vi "main(Test DQMH modules).vi"() -> ()   [LabVIEW 2018, in "Application.lvlib"]
uses:
  Application.lvlib
  eMIC response.ctl
  DRV stand.ctl
  type defs/HW config.ctl
  eMICs Cluster.ctl
  SubVIs/App state data.ctl
  SubVIs/Trigger cluster.ctl
  type defs/DMM all config cluster.ctl
  type defs/DMM config cluster.ctl
  SubVIs/FGV DRV data.ctl
  SubVIs/DUT data Mode.ctl
  Instrument Drivers/LV_driver_MBrelay/type defs/FGV enum.ctl
  SubVIs/Step data.ctl
  DRV cluster 2.ctl
  <vilib>/ErrorRing/Error Ring.xnode
  Switches Module/MB switches Module.lvlib
  MB 01 switches Module/MB 01 switches Module.lvlib
  DMM Module/DMM Module.lvlib
  v2_CE14/CE14_v2.lvlib
  Instrument Drivers/LV_driver_MBrelay/MB Relay.lvlib
panel:
  out "PCB":string
  out "Report file Name":string
  in  "RE_Test":bool caption="Again"
  in  "milliseconds to wait":u32=1500
  in  "Log report":bool
  in  "10-1 delay":u32=70
  in  "6_1 delay2":u32=70
  in  "DMM delay":u32=10
  in  "6_1 delay":u32=150
  in  "1-10delay":u32=70
  in  "eMIC delay":u32=70
  in  "DRV number":u8=1 max=60
  in  "Test Single DRV":bool
  in  "Enum":T1(ring)=enum."Fixxed"
  out "Name":string
  out "SAP ID":string
  out "Progress":string
  out "DRV stand":T2
  in  "Auto/Man":bool
  out "DC Measure Completed":bool caption="DC Completed"
  in  "Test Channel 10":bool
  in  "Test Channel 9":bool
  in  "Test Channel 8":bool
  in  "Test Channel 7":bool
  in  "Test Channel 6":bool
  in  "Test Channel 5":bool
  in  "Test Channel 4":bool
  in  "Test Channel 3":bool
  in  "Test Channel 2":bool
  in  "Test Channel 1":bool
  in  "Shorted Circuits Test":bool
  out "CE14  Module did it":bool[](array[boolean])
  out "time elased(ms)":u32
  out "Inst. 9":bool
  in  "Exit":bool
  out "Inst. 8":bool
  out "Inst. 7":bool
  out "Inst. 6":bool
  out "Inst. 5":bool
  out "Inst. 4":bool
  out "Inst. 3":bool
  out "Inst. 2":bool
  out "Inst. 1":bool
  out "new Trigger?":bool
  out "last Trigger?":bool
  out "error out":errorcluster
  out "State log":string
  out "AC  Completed":bool caption="AC Completed"
  in  "Select CE14 eMIC Module Instance":i32(ring)=-1 items=["All"=-1, "1"=1, "2"=2, "3"=3, "4"=4, "5"=5, "6"=6]
  out "New board?":bool
  in  "Test":bool caption="Again"
  out "DRV 61":u32(colorbox)
  in  "Settings":bool
  in  "VIEW":bool caption="Again"
  out "DRV 60":u32(colorbox) caption="60"
  out "DRV 59":u32(colorbox) caption="59"
  out "DRV 58":u32(colorbox) caption="58"
  out "DRV 57":u32(colorbox) caption="57"
  out "DRV 56":u32(colorbox) caption="56"
  out "DRV 55":u32(colorbox) caption="55"
  out "DRV 54":u32(colorbox) caption="54"
  out "DRV 53":u32(colorbox) caption="53"
  out "DRV 52":u32(colorbox) caption="52"
  out "DRV 51":u32(colorbox) caption="51"
  out "DRV 50":u32(colorbox) caption="50"
  out "DRV 49":u32(colorbox) caption="49"
  out "DRV 48":u32(colorbox) caption="48"
  out "DRV 47":u32(colorbox) caption="47"
  out "DRV 46":u32(colorbox) caption="46"
  out "DRV 45":u32(colorbox) caption="45"
  out "DRV 44":u32(colorbox) caption="44"
  out "DRV 43":u32(colorbox) caption="43"
  out "DRV 42":u32(colorbox) caption="42"
  out "DRV 41":u32(colorbox) caption="41"
  out "DRV 40":u32(colorbox) caption="40"
  out "DRV 39":u32(colorbox) caption="39"
  out "DRV 38":u32(colorbox) caption="38"
  out "DRV 37":u32(colorbox) caption="37"
  out "DRV 36":u32(colorbox) caption="36"
  out "DRV 35":u32(colorbox) caption="35"
  out "DRV 34":u32(colorbox) caption="34"
  out "DRV 33":u32(colorbox) caption="33"
  out "DRV 32":u32(colorbox) caption="32"
  out "DRV 31":u32(colorbox) caption="31"
  out "DRV 30":u32(colorbox) caption="30"
  out "DRV 29":u32(colorbox) caption="29"
  out "DRV 28":u32(colorbox) caption="28"
  out "DRV 27":u32(colorbox) caption="27"
  out "DRV 26":u32(colorbox) caption="26"
  out "DRV 25":u32(colorbox) caption="25"
  out "DRV 24":u32(colorbox) caption="24"
  out "DRV 23":u32(colorbox) caption="23"
  out "DRV 22":u32(colorbox) caption="22"
  out "DRV 21":u32(colorbox) caption="21"
  out "DRV 20":u32(colorbox) caption="20"
  out "DRV 19":u32(colorbox) caption="19"
  out "DRV 18":u32(colorbox) caption="18"
  out "DRV 17":u32(colorbox) caption="17"
  out "DRV 16":u32(colorbox) caption="16"
  out "DRV 15":u32(colorbox) caption="15"
  out "DRV 14":u32(colorbox) caption="14"
  out "DRV 13":u32(colorbox) caption="13"
  out "DRV 12":u32(colorbox) caption="12"
  out "DRV 11":u32(colorbox) caption="11"
  out "DRV 10":u32(colorbox) caption="10"
  out "DRV 9":u32(colorbox) caption="9"
  out "DRV 8":u32(colorbox) caption="8"
  out "DRV 7":u32(colorbox) caption="7"
  out "DRV 6":u32(colorbox) caption="6"
  out "DRV 5":u32(colorbox) caption="5"
  out "DRV 4":u32(colorbox) caption="4"
  out "DRV 3":u32(colorbox) caption="3"
  out "DRV 2":u32(colorbox) caption="2"
  out "DRV 1":u32(colorbox) caption="1"
  out "version":string caption="Version"
  out "Module ID":i32
  in  "Tab Control":T3(tab)
  out "Short DRV":bool[][](array[boolean])
  in  "Mux 10-1":bool
  in  "mux 6-1":bool
  in  "Read Optos":bool
  in  "Select DMM's Current Input":bool
  in  "mux2-1(DMM I) encode":enum16{"DMM I (0.5)", "DMM I (12)"}(ring)
  in  "mux 6-1 data":T4(ring)
  in  "mux 10-1 data":T5(ring)
  in  "set value":bool
  in  "Set trigger value":bool
  out "trigger Value":bool
  in  "Read trigger":bool
  in  "Reset JIG":bool
  in  "eMIC":bool
  in  "DEMUX 1-10":bool
  in  "TurnON/OFF +5V":bool
  in  "5V Value":bool
  in  "demux1_10(x6)_encode":T6(ring)
  in  "eMIC 6 values":bool[](array[boolean])=[FALSE, FALSE, FALSE, FALSE, FALSE, FALSE]
  in  "DMM query":bool
  in  "connect DMM":bool
  in  "DMM read dual value":bool
  in  "config DMM":bool
  in  "Detector Rate":u8(ring)=2 items=["SLOW", "MID", "FAST"]
  in  "DCI range":dbl=0.5
  in  "DCV range":dbl=1000.0
  out "DCV(Volts)":dbl
  out "DCI(mA)":dbl
  out "DMM func?":string
  out "DMM range?":string
  in  "request AC-all":bool
  in  "Open COM eMIC":bool
  in  "check connected":bool
  out "eMIC 1":T7
  out "eMIC 2":T7
  out "eMIC 3":T7
  out "eMIC 4":T7
  out "eMIC 5":T7
  out "eMIC 6":T7
  out "EMIC connected":bool[](array[boolean])
  out "AC switches Module":bool
  out "DC Measure Module":bool
  out "DC Switches Module":bool
  out "AC Measure Module":bool
  # "HV-60D: ON-LINE TESTER FOR LED POWER DRIVER"
  # "60"
  # "6"
  # "12"
  # "18"
  # "24"
  # "30"
  # "36"
  # "42"
  # "48"
  # "54"
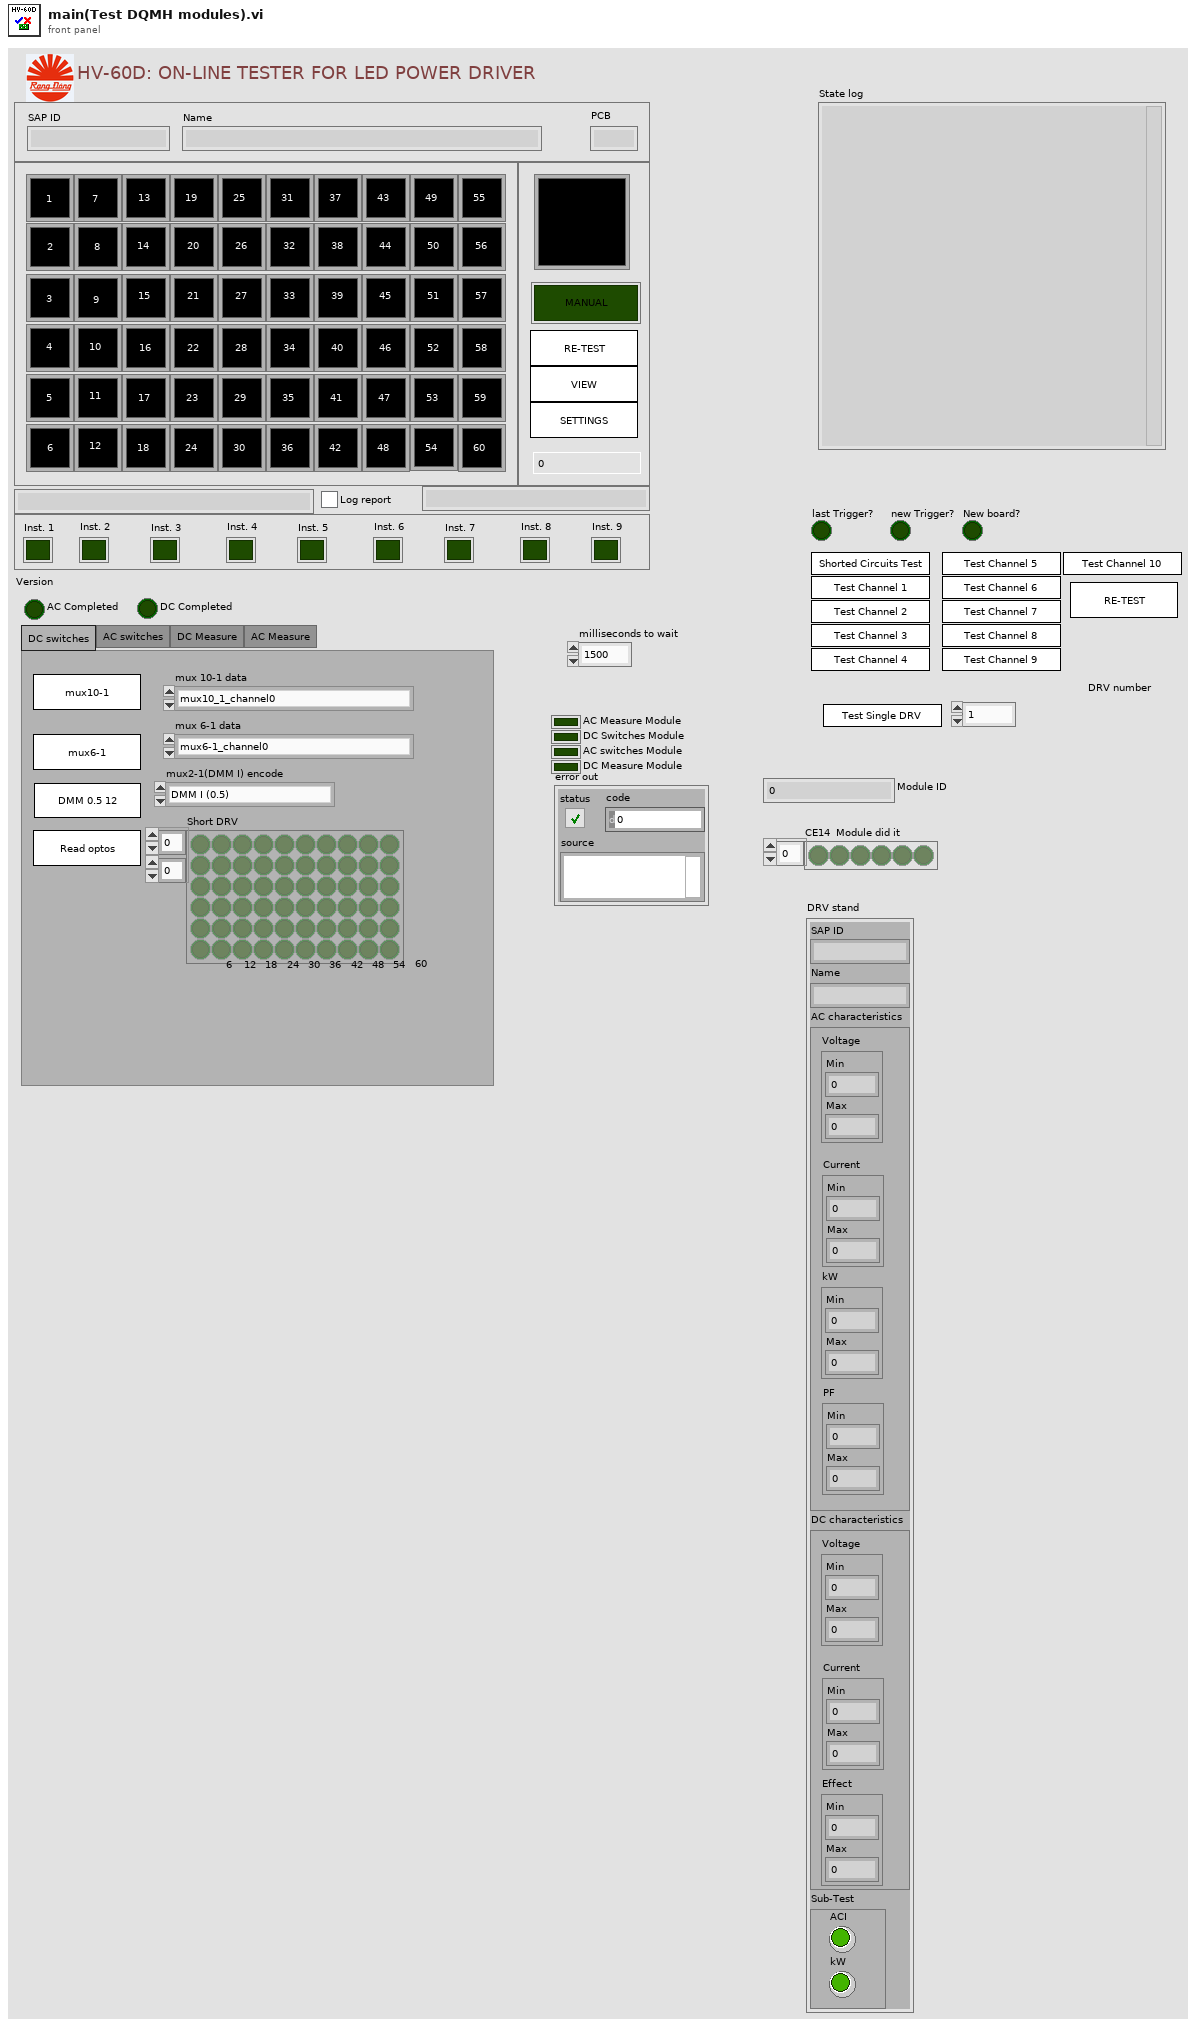
[diagram p1: front panel]
types:
  T1 = enum16{"All DRV", "Fixxed", "Pinpoint_JIG", "00037845(M26)"}
  T2 = typedef "Application.lvlib/DRV stand.ctl" = cluster{"SAP ID":string, "Name":string, "AC characteristics":cluster{"Voltage":cluster{"Min":dbl, "Max":dbl}, "Current":cluster{"Min":dbl, "Max":dbl}, "kW":cluster{"Min":dbl, "Max":dbl}, "PF":cluster{"Min":dbl, "Max":dbl}}, "DC characteristics":cluster{"Voltage":cluster{"Min":dbl, "Max":dbl}, "Current":cluster{"Min":dbl, "Max":dbl}, "Effect":cluster{"Min":dbl, "Max":dbl}}, "Sub-Test":cluster{"ACV":bool, "ACI":bool, "kW":bool, "PF":bool, "DCV":bool, "DCI":bool, "efficiency":bool}}
  T3 = enum32{"DC switches", "AC switches", "DC Measure", "AC Measure"}
  T4 = enum16{"mux6-1_channel0", "mux6_1_channel1_0", "mux6_1_channel1_1", "mux6-1_channel1_2", "mux6_1_channel1_3", "mux6_1_channel2_0", "mux6_1_channel2_1", "mux6_1_channel2_2", "mux6_1_channel2_3", "mux6_1_channel3_0", "mux6_1_channel3_1", "mux6_1_channel3_2", "mux6_1_channel3_3", "mux6_1_channel4_0", "mux6_1_channel4_1", "mux6_1_channel4_2", "mux6_1_channel4_3", "mux6_1_channel5_0", "mux6_1_channel5_1", "mux6_1_channel5_2", "mux6_1_channel5_3", "mux6_1_channel6_0", "mux6_1_channel6_1", "mux6_1_channel6_2", "mux6_1_channel6_3"}
  T5 = enum16{"mux10_1_channel0", "mux10_1_channel1", "mux10_1_channel2", "mux10_1_channel3", "mux10_1_channel4", "mux10_1_channel5", "mux10_1_channel6", "mux10_1_channel7", "mux10_1_channel8", "mux10_1_channel9", "mux10_1_channel10"}
  T6 = enum16{"demux1_10_channel0", "demux1_10_channel1", "demux1_10_channel2", "demux1_10_channel3", "demux1_10_channel4", "demux1_10_channel5", "demux1_10_channel6", "demux1_10_channel7", "demux1_10_channel8", "demux1_10_channel9", "demux1_10_channel10"}
  T7 = typedef "Application.lvlib/eMIC response.ctl" = cluster{"ACV":dbl, "ACI":dbl, "pF":dbl, "kW":dbl, "Freq":dbl, "kvar":dbl}
  T8 = typedef "Application.lvlib/eMICs Cluster.ctl" = cluster{"eMIC 1":T7, "eMIC 2":T7, "eMIC 3":T7, "eMIC 4":T7, "eMIC 5":T7, "eMIC 6":T7}
  T9 = typedef "Application.lvlib/HW config.ctl" = cluster{"DMM":string, "mux":string, "demux":string, "eMIC1":string, "eMIC2":string, "eMIC3":string, "eMIC4":string, "eMIC5":string, "eMIC6":string}
  T10 = typedef "Application.lvlib/Trigger cluster.ctl" = cluster{"new board?":bool, "new trigger":bool, "last trigger":bool}
  T11 = typedef "Application.lvlib/App state data.ctl" = cluster{"command":string, "command data":variant}
  T12 = typedef "CE14_v2.lvlib/Broadcast Events--cluster.ctl" = cluster{"Module Did Init":refnum<user-event>, "Status Updated":refnum<user-event>, "Error Reported":refnum<user-event>, "Module Did Stop":refnum<user-event>, "Update Module Execution Status":refnum<user-event>, "CE14 response data":refnum<user-event>}
  T13 = typedef "MB switches Module.lvlib/Broadcast Events--cluster.ctl" = cluster{"Module Did Init":refnum<user-event>, "Status Updated":refnum<user-event>, "Error Reported":refnum<user-event>, "Module Did Stop":refnum<user-event>, "Update Module Execution Status":refnum<user-event>}
  T14 = typedef "MB 01 switches Module.lvlib/Broadcast Events--cluster.ctl" = cluster{"Module Did Init":refnum<user-event>, "Status Updated":refnum<user-event>, "Error Reported":refnum<user-event>, "Module Did Stop":refnum<user-event>, "Update Module Execution Status":refnum<user-event>}
  T15 = typedef "DMM Module.lvlib/Broadcast Events--cluster.ctl" = cluster{"Module Did Init":refnum<user-event>, "Status Updated":refnum<user-event>, "Error Reported":refnum<user-event>, "Module Did Stop":refnum<user-event>, "Update Module Execution Status":refnum<user-event>}
  T16 = enum16{"open", "replace", "create", "open or create", "replace or create", "replace or create with confirmation"}
  T17 = typedef "Application.lvlib/DRV cluster 2.ctl" = cluster{"Shorted Circuit":bool, "AC voltage(volts)":dbl, "AC Current (mA)":dbl, "AC kW (W)":dbl, "AC pF ":dbl, "DC Voltage (Volts)":dbl, "DC Current (mA)":dbl, "DC kW (W)":dbl, "DRV Fail/Pass (T)":bool, "efficient (%)":dbl}
  T18 = enum32{"Invalid", "Standard", "Closed", "Hidden", "Minimized", "Maximized"}
  T19 = typedef "Application.lvlib/DMM all config cluster.ctl" = cluster{"DMM config cluster":T20, "mux2-1(DMM I) encode":enum16{"DMM I (0.5)", "DMM I (12)"}}
  T20 = typedef "Application.lvlib/DMM config cluster.ctl" = cluster{"DCV range":dbl, "DCI range":dbl, "Detector Rate":u8}
  T21 = typedef "Application.lvlib/DUT data Mode.ctl" = enum16{"range Limit", "Short Circuits", "AC parameter", "AC parameter 1", "DC parameter"}
  T22 = typedef "Application.lvlib/FGV DRV data.ctl" = enum16{"Init", "Write", "Read", "Process"}
  T23 = typedef "MB Relay.lvlib/FGV enum.ctl" = enum16{"Write", "Init FGV", "Read", "All OFF", "All ON"}
  T24 = typedef "CE14_eMIC.lvlib/CE14.data.ctl" = cluster{"string":string, "float":dbl, "Name":string}
  T25 = typedef "Application.lvlib/Step data.ctl" = cluster{"command":string, "Data":variant}
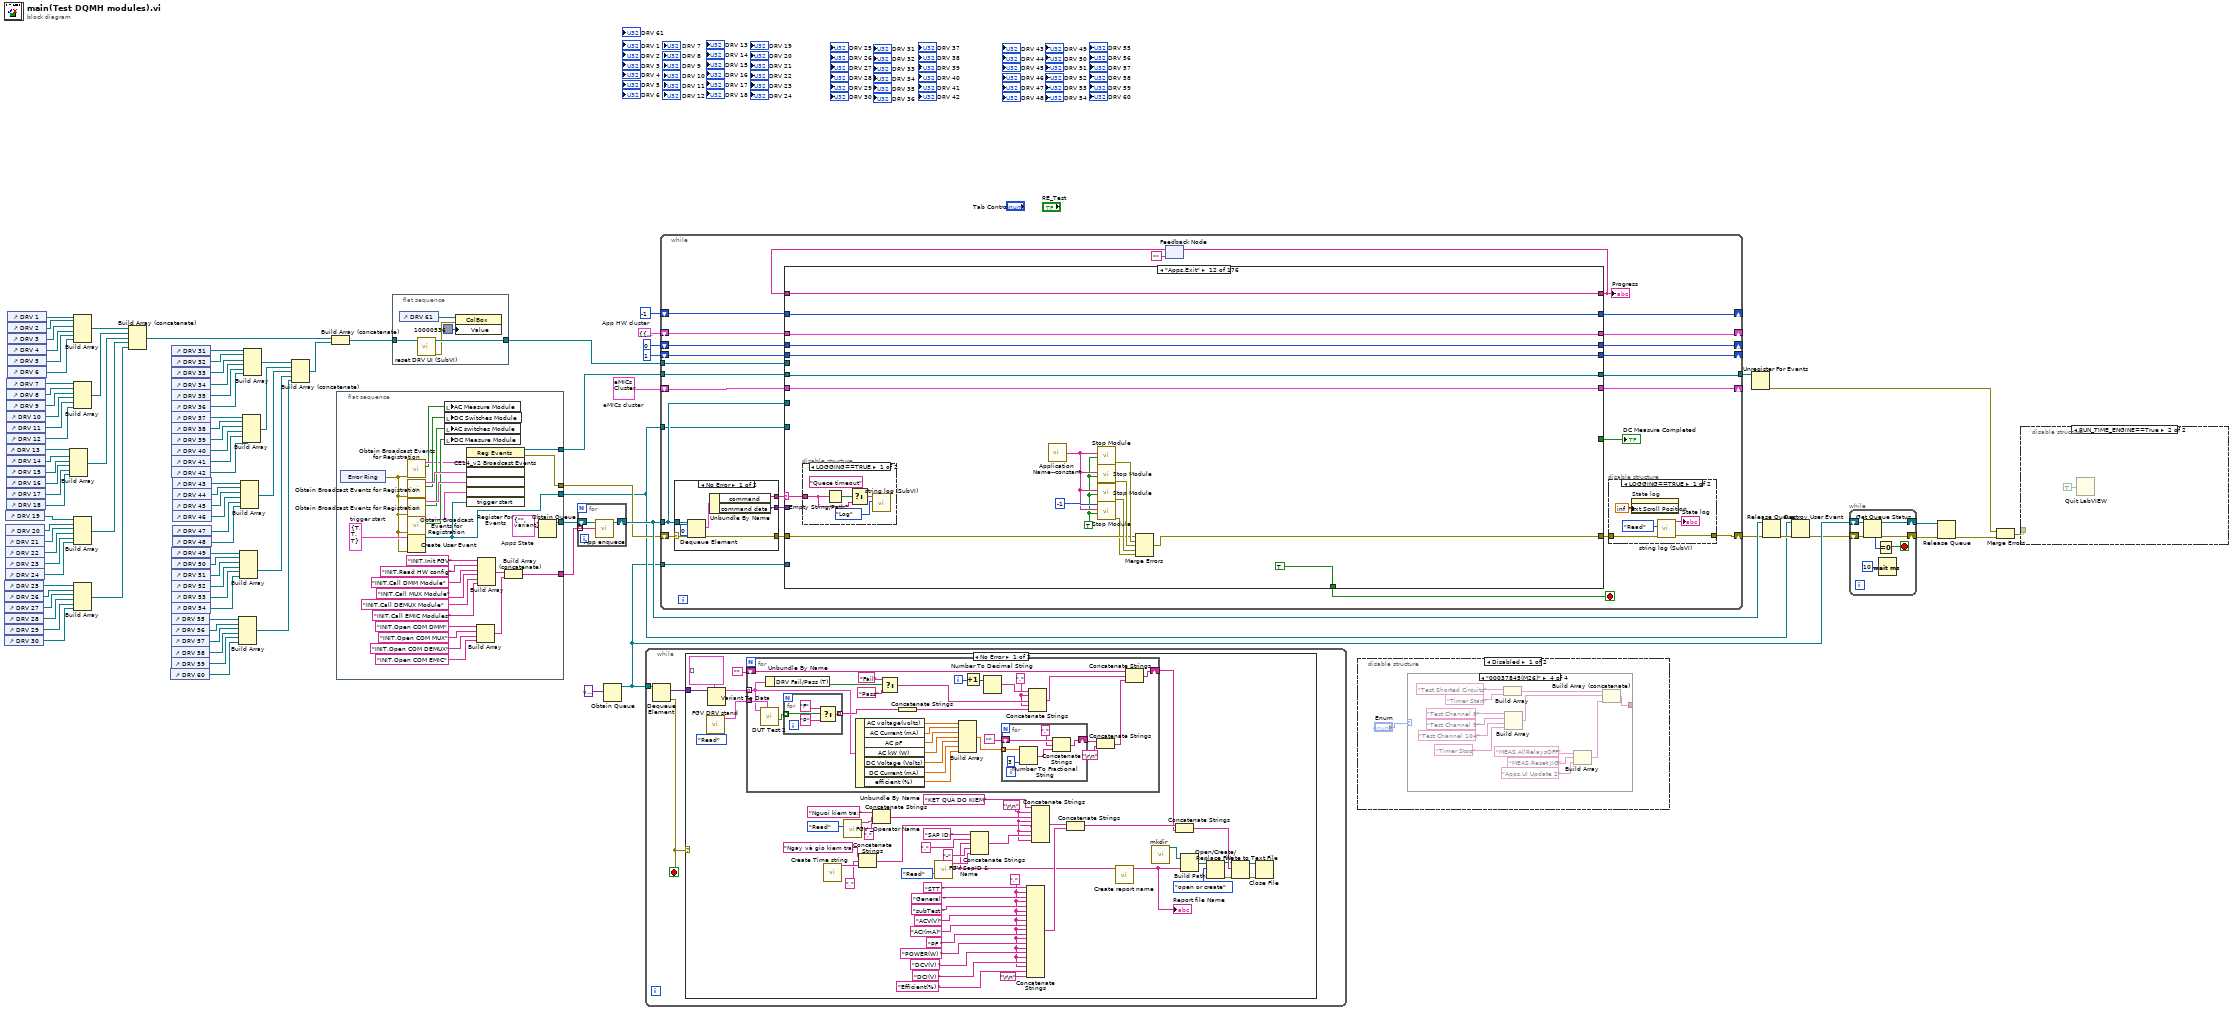
[diagram p0: block diagram]
diagram:
  w88 = T8 {"eMIC 1"={"ACV"=0.0, "ACI"=0.0, "pF"=0.0, "kW"=0.0, "Freq"=0.0, "kvar"=0.0}, "eMIC 2"={"ACV"=0.0, "ACI"=0.0, "pF"=0.0, "kW"=0.0, "Freq"=0.0, "kvar"=0.0}, "eMIC 3"={"ACV"=0.0, "ACI"=0.0, "pF"=0.0, "kW"=0.0, "Freq"=0.0, "kvar"=0.0}, "eMIC 4"={"ACV"=0.0, "ACI"=0.0, "pF"=0.0, "kW"=0.0, "Freq"=0.0, "kvar"=0.0}, "eMIC 5"={"ACV"=0.0, "ACI"=0.0, "pF"=0.0, "kW"=0.0, "Freq"=0.0, "kvar"=0.0}, "eMIC 6"={"ACV"=0.0, "ACI"=0.0, "pF"=0.0, "kW"=0.0, "Freq"=0.0, "kvar"=0.0}}  # eMICs cluster
  w93 = cluster{"HW config 2":T9} {"HW config 2"={"DMM"="COM15", "mux"="COM11", "demux"="COM16", "eMIC1"="COM13", "eMIC2"="COM6", "eMIC3"="COM9", "eMIC4"="COM10", "eMIC5"="COM12", "eMIC6"="COM11"}}  # App HW cluster
  n1 = control-ref of="DRV 25"() -> (w58:refnum<vi>)
  n2 = control-ref of="DRV 26"() -> (w59:refnum<vi>)
  n3 = control-ref of="DRV 27"() -> (w60:refnum<vi>)
  n4 = control-ref of="DRV 28"() -> (w61:refnum<vi>)
  n5 = control-ref of="DRV 29"() -> (w62:refnum<vi>)
  n6 = control-ref of="DRV 30"() -> (w63:refnum<vi>)
  n7 = control-ref of="DRV 21"() -> (w67:refnum<vi>)
  n8 = control-ref of="DRV 22"() -> (w66:refnum<vi>)
  n9 = control-ref of="DRV 23"() -> (w65:refnum<vi>)
  n10 = control-ref of="DRV 24"() -> (w64:refnum<vi>)
  n11 = control-ref of="DRV 19"() -> (w69:refnum<vi>)
  n12 = control-ref of="DRV 20"() -> (w68:refnum<vi>)
  n13 = control-ref of="DRV 13"() -> (w75:refnum<vi>)
  n14 = control-ref of="DRV 7"() -> (w81:refnum<vi>)
  n15 = control-ref of="DRV 8"() -> (w80:refnum<vi>)
  n16 = control-ref of="DRV 9"() -> (w79:refnum<vi>)
  n17 = control-ref of="DRV 10"() -> (w78:refnum<vi>)
  n18 = control-ref of="DRV 11"() -> (w77:refnum<vi>)
  n19 = control-ref of="DRV 12"() -> (w76:refnum<vi>)
  n20 = control-ref of="DRV 14"() -> (w74:refnum<vi>)
  n21 = control-ref of="DRV 15"() -> (w73:refnum<vi>)
  n22 = control-ref of="DRV 16"() -> (w72:refnum<vi>)
  n23 = control-ref of="DRV 17"() -> (w71:refnum<vi>)
  n24 = control-ref of="DRV 18"() -> (w70:refnum<vi>)
  n25 = control-ref of="DRV 1"() -> (w87:refnum<vi>)
  n26 = control-ref of="DRV 2"() -> (w86:refnum<vi>)
  n27 = control-ref of="DRV 3"() -> (w85:refnum<vi>)
  n28 = control-ref of="DRV 4"() -> (w84:refnum<vi>)
  n29 = control-ref of="DRV 5"() -> (w83:refnum<vi>)
  n30 = control-ref of="DRV 6"() -> (w82:refnum<vi>)
  n31 = Build Array(w75, w74, w73, w72, w71, w70) -> (w55:refnum<vi>[])
  n32 = Build Array(w87, w86, w85, w84, w83, w82) -> (w57:refnum<vi>[])
  n33 = Build Array(w69, w68, w67, w66, w65, w64) -> (w54:refnum<vi>[])
  n34 = Build Array(w58, w59, w60, w61, w62, w63) -> (w53:refnum<vi>[])
  n35 = Build Array(w81, w80, w79, w78, w77, w76) -> (w56:refnum<vi>[])
  n36 = Build Array (concatenate)(w57, w56, w55, w54, w53) -> (w17:refnum<vi>[])
  n37 = control-ref of="DRV 60"() -> (w28:refnum<vi>)
  n38 = control-ref of="DRV 55"() -> (w23:refnum<vi>)
  n39 = control-ref of="DRV 56"() -> (w24:refnum<vi>)
  n40 = control-ref of="DRV 57"() -> (w25:refnum<vi>)
  n41 = control-ref of="DRV 58"() -> (w26:refnum<vi>)
  n42 = control-ref of="DRV 59"() -> (w27:refnum<vi>)
  n43 = control-ref of="DRV 31"() -> (w47:refnum<vi>)
  n44 = control-ref of="DRV 32"() -> (w48:refnum<vi>)
  n45 = control-ref of="DRV 33"() -> (w49:refnum<vi>)
  n46 = control-ref of="DRV 34"() -> (w50:refnum<vi>)
  n47 = control-ref of="DRV 35"() -> (w51:refnum<vi>)
  n48 = control-ref of="DRV 36"() -> (w52:refnum<vi>)
  n49 = control-ref of="DRV 37"() -> (w46:refnum<vi>)
  n50 = control-ref of="DRV 38"() -> (w45:refnum<vi>)
  n51 = control-ref of="DRV 39"() -> (w44:refnum<vi>)
  n52 = control-ref of="DRV 40"() -> (w43:refnum<vi>)
  n53 = control-ref of="DRV 41"() -> (w42:refnum<vi>)
  n54 = control-ref of="DRV 42"() -> (w41:refnum<vi>)
  n55 = control-ref of="DRV 49"() -> (w34:refnum<vi>)
  n56 = control-ref of="DRV 50"() -> (w33:refnum<vi>)
  n57 = control-ref of="DRV 51"() -> (w32:refnum<vi>)
  n58 = control-ref of="DRV 52"() -> (w31:refnum<vi>)
  n59 = control-ref of="DRV 53"() -> (w30:refnum<vi>)
  n60 = control-ref of="DRV 54"() -> (w29:refnum<vi>)
  n61 = control-ref of="DRV 43"() -> (w35:refnum<vi>)
  n62 = control-ref of="DRV 44"() -> (w36:refnum<vi>)
  n63 = control-ref of="DRV 45"() -> (w37:refnum<vi>)
  n64 = control-ref of="DRV 46"() -> (w38:refnum<vi>)
  n65 = control-ref of="DRV 47"() -> (w39:refnum<vi>)
  n66 = control-ref of="DRV 48"() -> (w40:refnum<vi>)
  n67 = Build Array(w23, w24, w25, w26, w27, w28) -> (w18:refnum<vi>[])
  n68 = Build Array(w34, w33, w32, w31, w30, w29) -> (w19:refnum<vi>[])
  n69 = Build Array(w35, w36, w37, w38, w39, w40) -> (w20:refnum<vi>[])
  n70 = Build Array(w46, w45, w44, w43, w42, w41) -> (w21:refnum<vi>[])
  n71 = Build Array(w47, w48, w49, w50, w51, w52) -> (w22:refnum<vi>[])
  n72 = Build Array (concatenate)(w22, w21, w20, w19, w18) -> (w16:refnum<vi>[])
  n73 = Build Array (concatenate)(w17, w16) -> (w14:refnum<vi>[])
  n74 = flat-sequence {
    tunnel: [w118] -> w95
    tunnel: [w117] -> w92
    tunnel: [w116] -> w91
    tunnel: [w115] -> w15
    tunnel: [w110] -> w7
    frame #0 {
      w111 = T10 {"new board?"=TRUE, "new trigger"=TRUE, "last trigger"=TRUE}  # trigger start
      w112 = T11 {"command"="", "command data"=variant}  # Apps State
      n75 = xnode "Error Ring"() -> ("error out"=w109:errorcluster)
      n76 = call "Obtain Broadcast Events for Registration.vi"("error in (no error)"=w109) -> ("Already running?"=w113:bool, "CE14_v2 Broadcast Events"=w114:T12)  [unwired: 8 in, 1 out]
      n77 = call "Obtain Broadcast Events for Registration.vi"("error in (no error)"=w109) -> ("Already running?"=w121:bool, "Switches Module Broadcast Events"=w124:T13)  [unwired: 8 in, 1 out]
      n78 = call "Obtain Broadcast Events for Registration.vi"("error in (no error)"=w109) -> ("Already running?"=w120:bool, "MB 01 switches Module Broadcast Events"=w123:T14)  [unwired: 8 in, 1 out]
      n79 = call "Obtain Broadcast Events for Registration.vi"("error in (no error)"=w109) -> ("Already running?"=w119:bool, "DMM Module Broadcast Events"=w122:T15)  [unwired: 8 in, 1 out]
      n80 = Create User Event(user event datatype=w111, error in=w109) -> (user event=w110:refnum<user-event>)  [unwired: 1 out]
      n81 = local write "AC Measure Module"(w113) -> ()
      n82 = local write "DC Switches Module"(w121) -> ()
      n83 = local write "AC switches Module"(w120) -> ()
      n84 = local write "DC Measure Module"(w119) -> ()
      n85 = register-events(w114, w124, w123, w122, w110) -> (reference out=w118:refnum<event-registration>, error out=w115:errorcluster)  [unwired: 2 in]
      n86 = Build Array("INIT.Open COM DMM", "INIT.Open COM MUX", "INIT.Open COM DEMUX", "INIT.Open COM EMIC") -> (w106:string[])
      n87 = Build Array("INIT.Init FGV", "INIT.Read HW config", "INIT.Call DMM Module", "INIT.Call MUX Module", "INIT.Call DEMUX Module", "INIT.Call EMIC Modules") -> (w107:string[])
      n88 = Build Array (concatenate)(w107, w106) -> (w116:string[])
      n89 = Obtain Queue(element data type=w112) -> (queue out=w117:refnum<queue>)  [unwired: 4 in, 2 out]
    }
  }
  n90 = flat-sequence {
    tunnel: w14 -> [w130]
    tunnel: [w129] -> w13
    frame #0 {
      n91 = control-ref of="DRV 61"() -> (w126:refnum<vi>)
      n92 = call "reset DRV UI (SubVI).vi"("Ref  in"=w130) -> ("error out"=w127:errorcluster, "Ref out"=w129:refnum<vi>[])  [unwired: 9 in]
      n93 = property class="ColBox"(reference=w126, error in=w127, "Value"=u32 10000536 ("DRV 1")) -> ()  [unwired: 2 out]
    }
  }
  n94 = for {
    tunnel: w91 -> [w133] mode=indexing
    shift-right: [w131] -> w90
    shift-left: w92 -> [w132]
    n95 = call "App enquece.vi"("command"=w133, "queue in"=w132) -> ("Queue out"=w131:refnum<queue>)  [unwired: 8 in, 1 out]
  }
  n96 = Obtain Queue(element data type=variant) -> (queue out=w5:refnum<queue>)  [unwired: 4 in, 2 out]
  n97 = while {
    tunnel: w5 -> [w136]
    stop <- w134 stop-if-true
    n98 = Dequeue Element(queue=w136) -> (element=w135:variant, error out=w134:errorcluster)  [unwired: 2 in, 2 out]
    n99 = case shown="No Error" w134 {
      tunnel: w135 -> [w184 _]
      frame No Error {
        w149 = ","
        w157 = "\r\n"
        n100 = call "FGV DRV stand.vi"("Enum"=enum16{"Write", "Read"}."Read" ("Enum 2")) -> ("DRV stand out"=w181:T2)  [unwired: 10 in]
        n101 = Variant To Data(type=T17[] [] ("60 DRV data"), Variant=w184) -> (data=w183:T17[])  [unwired: 1 in, 1 out]
        n102 = for {
          tunnel: w183 -> [w202] mode=indexing
          tunnel: w181 -> [w213]
          shift-right: [w190] -> w159
          shift-left: "" -> [w189]
          i -> [w207]
          w186 = ","
          n103 = call "DUT Test 2.vi"("DRV stand"=w213, "DRV data"=w202) -> ("actual subtest"=w209:bool[])  [unwired: 6 in, 3 out]
          n104 = Unbundle By Name(w202) -> ("DRV Fail/Pass (T)"=w212:bool)
          n105 = for {
            tunnel: w209 -> [w222] mode=indexing
            tunnel: [w221] -> w208 mode=indexing
            n106 = Select(t="F", s=w222, f="P") -> (s? t:f=w221:string)
          }
          n107 = Unbundle By Name(w202) -> ("AC voltage(volts)"=w201:dbl, "AC Current (mA)"=w200:dbl, "AC pF"=w199:dbl, "AC kW (W)"=w198:dbl, "DC Voltage (Volts)"=w197:dbl, "DC Current (mA)"=w196:dbl, "efficient (%)"=w195:dbl)
          n108 = Select(t="Fail", s=w212, f="Pass") -> (s? t:f=w204:string)
          n109 = Concatenate Strings(w208) -> (w203:string)
          n110 = Build Array(w201, w200, w199, w198, w197, w196, w195) -> (w194:dbl[])
          n111 = Increment(x=w207) -> (x+1=w206:i32)
          n112 = Number To Decimal String(number=w206) -> (decimal integer string=w205:string)  [unwired: 1 in]
          n113 = for {
            tunnel: w194 -> [w219] mode=indexing
            shift-right: [w216] -> w192
            shift-left: "" -> [w217]
            n114 = Number To Fractional String(number=w219, precision (6)=i16 3) -> (F-format string=w215:string)  [unwired: 2 in]
            n115 = Concatenate Strings(w217, ",", w215) -> (w216:string)
          }
          n116 = Concatenate Strings(w205, w186, w204, w186, w203) -> (w188:string)
          n117 = Concatenate Strings(w192, "\r\n") -> (w187:string)
          n118 = Concatenate Strings(w189, w188, w187) -> (w190:string)
        }
        n119 = call "Create Time string.vi"() -> ("Timestr"=w155:string)  [unwired: 10 in, 1 out]
        n120 = call "FGV _Operator Name.vi"("Enum"=enum16{"Write", "Read"}."Read") -> ("Operator Name out"=w179:string)  [unwired: 10 in]
        n121 = Concatenate Strings("Ngay và gio kiem tra:", ",", w155) -> (w154:string)
        n122 = Concatenate Strings("Nguoi kiem tra:", ",", w179) -> (w180:string)
        n123 = call "FGV SapID & Name.vi"("Enum"=enum16{"Read", "Write"}."Read") -> ("SAP ID out"=w139:string, "Name out"=w140:string)  [unwired: 9 in]
        n124 = Concatenate Strings("SAP ID:", ",", w139, "-", w140) -> (w158:string)
        n125 = Concatenate Strings("STT ", w149, "General ", w149, "subTest ", w149, "ACV(V)", w149, "ACI(mA)", w149, "PF ", w149, "POWER(W) ", w149, "DCV(V) ", w149, "DCI(V) ", w149, "Efficient(%) ", "\r\n") -> (w162:string)
        n126 = Concatenate Strings("KET QUA DO KIEM" ("string"), w157, w180, w157, w154, w157, w158, w157) -> (w161:string)
        n127 = Concatenate Strings(w161, w162) -> (w160:string)
        n128 = call "Create report name.vi"("SAP ID"=w139) -> ("filename"=w137:string)  [unwired: 9 in, 1 out]
        "Report file Name" <- w137
        n129 = call "mkdir.vi"() -> ("created path"=w148:path)  [unwired: 10 in, 1 out]
        n130 = Concatenate Strings(w160, w159) -> (w145:string)
        n131 = Build Path(base path=w148, name or relative path=w137) -> (appended path=w147:path)
        n132 = Open/Create/Replace File(file path (use dialog)=w147, operation (0:open)=T16."open or create") -> (refnum out=w144:refnum<file>, error out=w143:errorcluster)  [unwired: 4 in, 1 out]
        n133 = Write to Text File(file (use dialog)=w144, text=w145, error in=w143) -> (refnum out=w141:refnum<file>, error out=w142:errorcluster)  [unwired: 1 in, 1 out]
        n134 = Close File(refnum=w141, error in=w142) -> ()  [unwired: 2 out]
      }
      frame Error {
      }
    }
  }
  n135 = while {
    shift-right: [w228] -> w89
    shift-left: w15 -> [w250]
    shift-right: [w248] -> _
    shift-left: -1 -> [w247]
    tunnel: w95 -> [w246]
    tunnel: [w245] -> w94
    shift-right: [w243] -> _
    shift-left: w93 -> [w244]
    tunnel: w90 -> [w232]
    shift-right: [w241] -> _
    shift-left: w88 -> [w240]
    tunnel: w13 -> [w238]
    shift-right: [w237] -> _
    shift-left: 1 ("DUT channel (1-11)") -> [w236]
    shift-right: [w235] -> _
    shift-left: 0 ("DUT index(0-59)") -> [w234]
    tunnel: w7 -> [w231]
    tunnel: w5 -> [w224]
    stop <- w239 stop-if-true
    n136 = case shown="No Error" w250 {
      selector: w250 -> [w262 w263]
      tunnel: [w260 "Apps.Error Handler"] -> w233
      tunnel: [w261 w263] -> w249
      tunnel: [w259 _] -> w242
      tunnel: w232 -> [w258 _]
      frame No Error {
        n137 = Dequeue Element(queue=w258, timeout in ms (-1)=0, error in (no error)=w262) -> (element=w257:T11, error out=w261:errorcluster)  [unwired: 2 out]
        n138 = Unbundle By Name(w257) -> ("command"=w260:string, "command data"=w259:variant)
      }
      frame Error {
      }
    }
    n139 = feedback #1("") -> (w226:string)
    n140 = case shown="\"Apps.Exit\"" w233 {
      selector: w233 -> [w273 _ _ w1278 w1298 w1436 w1468 w1531 _ _ _ w1621 w1644 _ w1703 w1771 w1786 w1809 w1832 w1857 w1891 w1910 w1929 w1948 w1981 w2011 w2036 w2065 w2098 w2119 w2143 w2178 w2194 w2219 w2254 w2287 w2326 w2376 w2416 w2461 w2516 w2588 w2658 w2729 w2800 w2871 w2942 w3013 w3085 w3158 w3234 w3313 w3393 w3474 w3556 w3606 w3645 w3686 w3727 w3768 w3807 w3850 w3891 w3932 w3973 w4014 w4055 w4096 w4137 w4178 w4219 w4260 w4299 w4342 w4383 w4424 w4465 w4506 w4547 w4588 w4629 w4670 w4711 w4752 w4793 w4834 w4875 w4916 w4957 w4998 w5039 w5080 w5121 w5162 w5203 w5244 w5285 w5326 w5367 w5408 w5449 w5490 w5531 w5572 w5613 w5654 w5695 w5736 w5777 w5818 w5859 w5900 w5941 w5982 w6023 _ w6080 w6137 w6194 w6251 w6308 w6365 w6422 w6479 w6536 w6593 w6650 w6707 w6764 w6821 w6879 w6936 w6993 w7050 w7107 w7164 w7221 w7278 w7335 w7392 w7449 w7506 w7563 w7620 w7677 w7734 w7791 w7848 w7905 w7962 w8019 w8076 w8133 w8191 w8247 w8304 w8361 w8418 w8475 w8532 w8589 w8646 w8705 w8760 w8817 w8874 w8931 w8988 w9046 w9102 w9159 w9216 w9276 w9335 w9394 w9453]
      tunnel: w249 -> [w279 w1263 w1266 w1279 w1305 w1438 w1481 w1539 w1595 w1598 w1619 w1629 w1658 w1683 w1715 w1772 w1787 w1810 w1833 w1858 w1892 w1911 w1930 w1949 w1984 w2012 w2037 w2066 w2101 w2122 w2142 w2179 w2195 w2220 w2255 w2292 w2329 w2379 w2417 w2455 w2518 w2590 w2660 w2731 w2802 w2873 w2944 w3015 w3087 w3160 w3236 w3315 w3395 w3476 w3558 w3609 w3650 w3691 w3732 w3773 w3814 w3855 w3896 w3937 w3978 w4019 w4060 w4101 w4142 w4183 w4224 w4265 w4306 w4347 w4388 w4429 w4470 w4511 w4552 w4593 w4634 w4675 w4716 w4757 w4798 w4839 w4880 w4921 w4962 w5003 w5044 w5085 w5126 w5167 w5208 w5249 w5290 w5331 w5372 w5413 w5454 w5495 w5536 w5577 w5618 w5659 w5700 w5741 w5782 w5823 w5864 w5905 w5946 w5987 w6028 w6069 w6086 w6143 w6200 w6257 w6314 w6371 w6428 w6485 w6542 w6599 w6656 w6713 w6770 w6827 w6885 w6942 w6999 w7056 w7113 w7170 w7227 w7284 w7341 w7398 w7455 w7512 w7569 w7626 w7683 w7740 w7797 w7854 w7911 w7968 w8025 w8082 w8139 w8196 w8253 w8310 w8367 w8424 w8481 w8538 w8595 w8652 w8697 w8766 w8823 w8880 w8937 w8994 w9052 w9108 w9165 w9222 w9282 w9341 w9400 w9459]
      tunnel: [w280 w1263 w1267 w1280 w1306 w1439 w1462 w1530 w1595 w1597 w1619 w1630 w1646 w1673 w1706 w1762 w1788 w1811 w1834 w1856 w1890 w1909 w1928 w1947 w1973 w2010 w2034 w2062 w2100 w2121 w2145 w2174 w2199 w2222 w2258 w2290 w2328 w2377 w2415 w2449 w2519 w2591 w2661 w2732 w2803 w2874 w2945 w3016 w3088 w3161 w3237 w3316 w3396 w3477 w3559 w3610 w3651 w3692 w3733 w3774 w3815 w3856 w3897 w3938 w3979 w4020 w4061 w4102 w4143 w4184 w4225 w4266 w4307 w4348 w4389 w4430 w4471 w4512 w4553 w4594 w4635 w4676 w4717 w4758 w4799 w4840 w4881 w4922 w4963 w5004 w5045 w5086 w5127 w5168 w5209 w5250 w5291 w5332 w5373 w5414 w5455 w5496 w5537 w5578 w5619 w5660 w5701 w5742 w5783 w5824 w5865 w5906 w5947 w5988 w6029 w6069 w6084 w6141 w6198 w6255 w6312 w6369 w6426 w6483 w6540 w6597 w6654 w6711 w6768 w6825 w6883 w6940 w6997 w7054 w7111 w7168 w7225 w7282 w7339 w7396 w7453 w7510 w7567 w7624 w7681 w7738 w7795 w7852 w7909 w7966 w8023 w8080 w8137 w8194 w8251 w8308 w8365 w8422 w8479 w8536 w8593 w8650 w8708 w8764 w8821 w8878 w8935 w8992 w9050 w9106 w9163 w9220 w9280 w9339 w9398 w9457] -> w229
      tunnel: [_ _ _ _ _ _ _ _ _ _ _ TRUE _ _ _ _ _ _ _ _ _ _ _ _ _ _ _ _ _ _ _ _ _ _ _ _ _ _ _ _ _ _ _ _ _ _ _ _ _ _ _ _ _ _ _ _ _ _ _ _ _ _ _ _ _ _ _ _ _ _ _ _ _ _ _ _ _ _ _ _ _ _ _ _ _ _ _ _ _ _ _ _ _ _ _ _ _ _ _ _ _ _ _ _ _ _ _ _ _ _ _ _ _ _ _ _ _ _ _ _ _ _ _ _ _ _ _ _ _ _ _ _ _ _ _ _ _ _ _ _ _ _ _ _ _ _ _ _ _ _ _ _ _ _ _ _ _ _ _ _ _ _ _ _ _ _ _ _ _ _ _ _ _ _ _ _] -> w239
      tunnel: [w284 100 w1276 w1289 w1309 w1442 w1463 w1538 w1594 w1606 w1618 w1636 w1657 w1682 w1714 w1779 w1802 w1825 w1848 w1872 w1899 w1918 w1937 w1957 w1990 w2026 w2045 w2072 w2089 w2132 w2151 w2175 w2206 w2230 w2273 w2298 w2337 w2387 w2422 w2479 w2538 w2609 w2680 w2751 w2822 w2893 w2964 w3035 w3106 w3177 w3253 w3332 w3412 w3493 w3575 w3615 w3656 w3697 w3738 w3779 w3820 w3861 w3902 w3943 w3984 w4025 w4066 w4107 w4148 w4189 w4230 w4271 w4312 w4353 w4394 w4435 w4476 w4517 w4558 w4599 w4640 w4681 w4722 w4763 w4804 w4845 w4886 w4927 w4968 w5009 w5050 w5091 w5132 w5173 w5214 w5255 w5296 w5337 w5378 w5419 w5460 w5501 w5542 w5583 w5624 w5665 w5706 w5747 w5788 w5829 w5870 w5911 w5952 w5993 w6034 w6068 w6116 w6173 w6230 w6287 w6344 w6401 w6458 w6515 w6572 w6629 w6686 w6743 w6800 w6857 w6914 w6971 w7028 w7085 w7142 w7199 w7256 w7313 w7370 w7427 w7484 w7541 w7598 w7655 w7712 w7769 w7826 w7883 w7940 w7997 w8054 w8111 w8168 w8225 w8282 w8339 w8396 w8453 w8510 w8567 w8624 w8681 w8738 w8795 w8852 w8909 w8966 w9023 w9080 w9137 w9194 w9251 w9310 w9369 w9428 w9487] -> w248
      tunnel: w247 -> [w272 _ w1276 w1289 w1309 w1442 w1463 w1538 w1594 w1606 w1618 w1636 w1657 w1682 w1714 w1779 w1802 w1825 w1848 w1872 w1899 w1918 w1937 w1957 w1990 w2026 w2045 w2072 w2088 w2132 w2151 w2175 w2206 w2230 w2273 w2298 w2337 w2387 w2422 w2479 w2538 w2609 w2680 w2751 w2822 w2893 w2964 w3035 w3106 w3177 w3253 w3332 w3412 w3493 w3575 w3615 w3656 w3697 w3738 w3779 w3820 w3861 w3902 w3943 w3984 w4025 w4066 w4107 w4148 w4189 w4230 w4271 w4312 w4353 w4394 w4435 w4476 w4517 w4558 w4599 w4640 w4681 w4722 w4763 w4804 w4845 w4886 w4927 w4968 w5009 w5050 w5091 w5132 w5173 w5214 w5255 w5296 w5337 w5378 w5419 w5460 w5501 w5542 w5583 w5624 w5665 w5706 w5747 w5788 w5829 w5870 w5911 w5952 w5993 w6034 w6068 w6116 w6173 w6230 w6287 w6344 w6401 w6458 w6515 w6572 w6629 w6686 w6743 w6800 w6857 w6914 w6971 w7028 w7085 w7142 w7199 w7256 w7313 w7370 w7427 w7484 w7541 w7598 w7655 w7712 w7769 w7826 w7883 w7940 w7997 w8054 w8111 w8168 w8225 w8282 w8339 w8396 w8453 w8510 w8567 w8624 w8681 w8738 w8795 w8852 w8909 w8966 w9023 w9080 w9137 w9194 w9251 w9310 w9369 w9428 w9487]
      tunnel: w246 -> [w283 w1262 w1275 w1288 w1308 w1441 w1480 w1537 w1593 w1605 w1617 w1635 w1656 w1681 w1713 w1778 w1800 w1823 w1846 w1865 w1898 w1917 w1936 w1956 w1989 w2025 w2044 w2071 w2107 w2131 w2150 w2185 w2205 w2229 w2272 w2297 w2336 w2386 w2421 w2478 w2537 w2608 w2679 w2750 w2821 w2892 w2963 w3034 w3068 w3176 w3252 w3331 w3411 w3492 w3574 w3614 w3655 w3696 w3737 w3778 w3819 w3860 w3901 w3942 w3983 w4024 w4065 w4106 w4147 w4188 w4229 w4270 w4311 w4352 w4393 w4434 w4475 w4516 w4557 w4598 w4639 w4680 w4721 w4762 w4803 w4844 w4885 w4926 w4967 w5008 w5049 w5090 w5131 w5172 w5213 w5254 w5295 w5336 w5377 w5418 w5459 w5500 w5541 w5582 w5623 w5664 w5705 w5746 w5787 w5828 w5869 w5910 w5951 w5992 w6033 w6067 w6115 w6172 w6229 w6286 w6343 w6400 w6457 w6514 w6571 w6628 w6685 w6742 w6799 w6856 w6913 w6970 w7027 w7084 w7141 w7198 w7255 w7312 w7369 w7426 w7483 w7540 w7597 w7654 w7711 w7768 w7825 w7882 w7939 w7996 w8053 w8110 w8167 w8224 w8281 w8338 w8395 w8452 w8509 w8566 w8623 w8680 w8737 w8794 w8851 w8908 w8965 w9022 w9079 w9136 w9193 w9250 w9309 w9368 w9427 w9486]
      tunnel: [w282 w1262 w1275 w1288 w1308 w1441 w1480 w1537 w1593 w1605 w1617 w1635 w1656 w1681 w1713 w1778 w1801 w1824 w1847 w1863 w1898 w1917 w1936 w1956 w1989 w2025 w2044 w2071 w2107 w2131 w2150 w2185 w2205 w2229 w2272 w2297 w2336 w2386 w2421 w2478 w2537 w2608 w2679 w2750 w2821 w2892 w2963 w3034 w3068 w3176 w3252 w3331 w3411 w3492 w3574 w3614 w3655 w3696 w3737 w3778 w3819 w3860 w3901 w3942 w3983 w4024 w4065 w4106 w4147 w4188 w4229 w4270 w4311 w4352 w4393 w4434 w4475 w4516 w4557 w4598 w4639 w4680 w4721 w4762 w4803 w4844 w4885 w4926 w4967 w5008 w5049 w5090 w5131 w5172 w5213 w5254 w5295 w5336 w5377 w5418 w5459 w5500 w5541 w5582 w5623 w5664 w5705 w5746 w5787 w5828 w5869 w5910 w5951 w5992 w6033 w6067 w6115 w6172 w6229 w6286 w6343 w6400 w6457 w6514 w6571 w6628 w6685 w6742 w6799 w6856 w6913 w6970 w7027 w7084 w7141 w7198 w7255 w7312 w7369 w7426 w7483 w7540 w7597 w7654 w7711 w7768 w7825 w7882 w7939 w7996 w8053 w8110 w8167 w8224 w8281 w8338 w8395 w8452 w8509 w8566 w8623 w8680 w8737 w8794 w8851 w8908 w8965 w9022 w9079 w9136 w9193 w9250 w9309 w9368 w9427 w9486] -> w245
      tunnel: w244 -> [w281 w1261 w1274 w1287 w1307 w1440 w1479 w1536 w1592 w1604 w1616 w1634 w1655 w1680 w1712 w1777 w1797 w1821 w1843 w1864 w1897 w1914 w1935 w1955 w1988 w2024 w2043 w2070 w2106 w2130 w2149 w2184 w2204 w2228 w2271 w2296 w2335 w2385 w2420 w2477 w2536 w2607 w2678 w2749 w2820 w2891 w2962 w3033 w3105 w3175 w3251 w3330 w3410 w3491 w3573 w3613 w3654 w3695 w3736 w3777 w3818 w3859 w3900 w3941 w3982 w4023 w4064 w4105 w4146 w4187 w4228 w4269 w4310 w4351 w4392 w4433 w4474 w4515 w4556 w4597 w4638 w4679 w4720 w4761 w4802 w4843 w4884 w4925 w4966 w5007 w5048 w5089 w5130 w5171 w5212 w5253 w5294 w5335 w5376 w5417 w5458 w5499 w5540 w5581 w5622 w5663 w5704 w5745 w5786 w5827 w5868 w5909 w5950 w5991 w6032 w6066 w6114 w6171 w6228 w6285 w6342 w6399 w6456 w6513 w6570 w6627 w6684 w6741 w6798 w6855 w6912 w6969 w7026 w7083 w7140 w7197 w7254 w7311 w7368 w7425 w7482 w7539 w7596 w7653 w7710 w7767 w7824 w7881 w7938 w7995 w8052 w8109 w8166 w8223 w8280 w8337 w8394 w8451 w8508 w8565 w8622 w8679 w8736 w8793 w8850 w8907 w8964 w9021 w9078 w9135 w9192 w9249 w9308 w9367 w9426 w9485]
      tunnel: [w281 w1261 w1274 w1287 w1307 w1440 w1479 w1536 w1592 w1604 w1616 w1634 w1655 w1680 w1710 w1777 w1797 w1821 w1843 w1864 w1897 w1914 w1935 w1955 w1988 w2024 w2043 w2070 w2106 w2130 w2149 w2184 w2204 w2228 w2271 w2296 w2335 w2385 w2420 w2477 w2536 w2607 w2678 w2749 w2820 w2891 w2962 w3033 w3105 w3175 w3251 w3330 w3410 w3491 w3573 w3613 w3654 w3695 w3736 w3777 w3818 w3859 w3900 w3941 w3982 w4023 w4064 w4105 w4146 w4187 w4228 w4269 w4310 w4351 w4392 w4433 w4474 w4515 w4556 w4597 w4638 w4679 w4720 w4761 w4802 w4843 w4884 w4925 w4966 w5007 w5048 w5089 w5130 w5171 w5212 w5253 w5294 w5335 w5376 w5417 w5458 w5499 w5540 w5581 w5622 w5663 w5704 w5745 w5786 w5827 w5868 w5909 w5950 w5991 w6032 w6066 w6114 w6171 w6228 w6285 w6342 w6399 w6456 w6513 w6570 w6627 w6684 w6741 w6798 w6855 w6912 w6969 w7026 w7083 w7140 w7197 w7254 w7311 w7368 w7425 w7482 w7539 w7596 w7653 w7710 w7767 w7824 w7881 w7938 w7995 w8052 w8109 w8166 w8223 w8280 w8337 w8394 w8451 w8508 w8565 w8622 w8679 w8736 w8793 w8850 w8907 w8964 w9021 w9078 w9135 w9192 w9249 w9308 w9367 w9426 w9485] -> w243
      tunnel: w242 -> [w265 _ _ _ w1296 _ _ _ _ _ w1609 _ _ _ _ _ _ _ _ _ _ _ _ _ _ w2023 _ _ _ w2127 _ _ w2203 w2227 w2270 w2285 w2334 w2384 _ _ _ _ _ _ _ _ _ _ _ _ _ _ _ _ _ _ _ _ _ _ _ _ _ _ _ _ _ _ _ _ _ _ _ _ _ _ _ _ _ _ _ _ _ _ _ _ _ _ _ _ _ _ _ _ _ _ _ _ _ _ _ _ _ _ _ _ _ _ _ _ _ _ _ _ _ _ _ _ _ _ _ _ _ _ _ _ _ _ _ _ _ _ _ _ _ _ _ _ _ _ _ _ _ _ _ _ _ _ _ _ _ _ _ _ _ _ _ _ _ _ _ _ _ _ _ _ _ _ _ _ _ _ _ _ _ _]
      tunnel: w232 -> [w278 _ w1270 w1286 _ _ w1460 _ _ _ _ _ w1652 _ w1700 w1764 _ _ _ _ _ _ _ _ w1968 _ _ _ _ _ _ _ _ _ _ _ _ _ _ w2467 w2503 w2573 w2644 w2714 w2786 w2856 w2929 w3000 w3071 w3144 w3223 w3301 w3382 w3463 w3546 w3608 w3649 w3690 w3731 w3772 w3813 w3854 w3895 w3936 w3977 w4018 w4059 w4100 w4141 w4182 w4223 w4264 w4305 w4346 w4387 w4428 w4469 w4510 w4551 w4592 w4633 w4674 w4715 w4756 w4797 w4838 w4879 w4920 w4961 w5002 w5043 w5084 w5125 w5166 w5207 w5248 w5289 w5330 w5371 w5412 w5453 w5494 w5535 w5576 w5617 w5658 w5699 w5740 w5781 w5822 w5863 w5904 w5945 w5986 w6027 _ w6081 w6138 w6195 w6252 w6309 w6366 w6423 w6480 w6537 w6594 w6651 w6708 w6765 w6822 w6880 w6937 w6994 w7051 w7108 w7165 w7222 w7279 w7336 w7393 w7450 w7507 w7564 w7621 w7678 w7735 w7792 w7849 w7906 w7963 w8020 w8077 w8134 w8192 w8248 w8305 w8362 w8419 w8476 w8533 w8590 w8647 w8706 w8761 w8818 w8875 w8932 w8989 w9047 w9103 w9160 w9217 w9277 w9336 w9395 w9454]
      tunnel: [w277 w1260 w1273 w1284 w1300 w1433 w1478 w1535 w1591 w1603 w1615 w1628 w1654 w1679 w1709 w1776 w1791 w1814 w1837 w1862 w1896 w1915 w1933 w1952 w1986 w2016 w2042 w2069 w2105 w2125 w2148 w2182 w2201 w2225 w2268 w2295 w2332 w2382 w2419 w2476 w2517 w2589 w2659 w2730 w2801 w2872 w2943 w3014 w3086 w3159 w3235 w3314 w3394 w3475 w3557 w3612 w3653 w3694 w3735 w3776 w3817 w3858 w3899 w3940 w3981 w4022 w4063 w4104 w4145 w4186 w4227 w4268 w4309 w4350 w4391 w4432 w4473 w4514 w4555 w4596 w4637 w4678 w4719 w4760 w4801 w4842 w4883 w4924 w4965 w5006 w5047 w5088 w5129 w5170 w5211 w5252 w5293 w5334 w5375 w5416 w5457 w5498 w5539 w5580 w5621 w5662 w5703 w5744 w5785 w5826 w5867 w5908 w5949 w5990 w6031 w6065 w6113 w6170 w6227 w6284 w6341 w6398 w6455 w6512 w6569 w6626 w6683 w6740 w6797 w6854 w6911 w6968 w7025 w7082 w7139 w7196 w7253 w7310 w7367 w7424 w7481 w7538 w7595 w7652 w7709 w7766 w7823 w7880 w7937 w7994 w8051 w8108 w8165 w8222 w8279 w8336 w8393 w8450 w8507 w8564 w8621 w8678 w8735 w8792 w8849 w8906 w8963 w9020 w9077 w9134 w9191 w9248 w9307 w9366 w9425 w9484] -> w241
      tunnel: w240 -> [w276 w1260 w1273 w1284 w1300 w1433 w1478 w1535 w1591 w1603 w1615 w1628 w1654 w1679 w1709 w1776 w1791 w1814 w1837 w1862 w1896 w1915 w1933 w1952 w1986 w2016 w2042 w2069 w2105 w2125 w2148 w2182 w2201 w2225 w2268 w2295 w2332 w2382 w2419 w2476 w2517 w2589 w2659 w2730 w2801 w2872 w2943 w3014 w3086 w3159 w3235 w3314 w3394 w3475 w3557 w3612 w3653 w3694 w3735 w3776 w3817 w3858 w3899 w3940 w3981 w4022 w4063 w4104 w4145 w4186 w4227 w4268 w4309 w4350 w4391 w4432 w4473 w4514 w4555 w4596 w4637 w4678 w4719 w4760 w4801 w4842 w4883 w4924 w4965 w5006 w5047 w5088 w5129 w5170 w5211 w5252 w5293 w5334 w5375 w5416 w5457 w5498 w5539 w5580 w5621 w5662 w5703 w5744 w5785 w5826 w5867 w5908 w5949 w5990 w6031 w6065 w6113 w6170 w6227 w6284 w6341 w6398 w6455 w6512 w6569 w6626 w6683 w6740 w6797 w6854 w6911 w6968 w7025 w7082 w7139 w7196 w7253 w7310 w7367 w7424 w7481 w7538 w7595 w7652 w7709 w7766 w7823 w7880 w7937 w7994 w8051 w8108 w8165 w8222 w8279 w8336 w8393 w8450 w8507 w8564 w8621 w8678 w8735 w8792 w8849 w8906 w8963 w9020 w9077 w9134 w9191 w9248 w9307 w9366 w9425 w9484]
      tunnel: w238 -> [w275 _ _ _ w1302 w1428 _ w1524 _ _ _ _ _ _ _ _ _ _ _ _ _ _ _ _ _ _ _ _ _ _ _ w2176 _ _ _ _ _ _ _ w2466 _ _ _ _ _ _ _ _ _ _ _ _ _ _ _ _ _ _ _ _ _ _ _ _ _ _ _ _ _ _ _ _ _ _ _ _ _ _ _ _ _ _ _ _ _ _ _ _ _ _ _ _ _ _ _ _ _ _ _ _ _ _ _ _ _ _ _ _ _ _ _ _ _ _ _ _ w6070 w6127 w6184 w6242 w6298 w6356 w6413 w6470 w6527 w6584 w6641 w6698 w6754 w6811 w6868 w6925 w6982 w7039 w7096 w7153 w7211 w7267 w7325 w7382 w7438 w7496 w7552 w7610 w7666 w7724 w7781 w7838 w7894 w7951 w8009 w8066 w8123 w8180 w8237 w8294 w8351 w8408 w8465 w8523 w8579 w8635 w8693 w8751 w8808 w8865 w8921 w8978 w9035 w9092 w9149 w9206 w9267 w9326 w9385 w9444]
